vi "创建配方子VI.vi"() -> (3 "配方编号":string)   [LabVIEW 2013]
panel:
  in  "确定":bool
  in  "配方编号":string
  # "请输入配方"
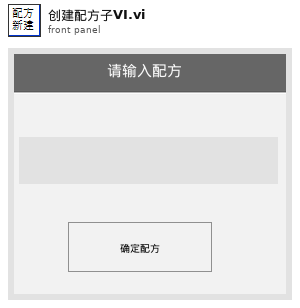
[diagram p1: front panel]
types:
  T1 = enum32{"Invalid", "Standard", "Closed", "Hidden", "Minimized", "Maximized"}
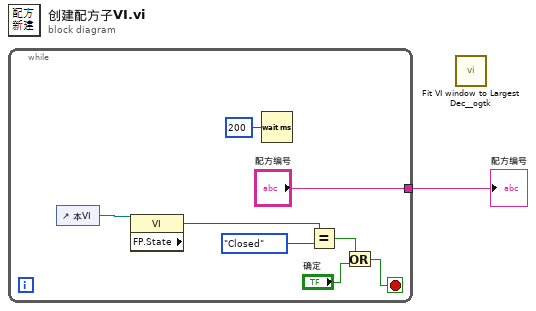
[diagram p0: block diagram]
diagram:
  n1 = while {
    tunnel: ["配方编号"] -> w1
    stop <- w2 stop-if-true
    n2 = control-ref of="本VI"() -> (w4:refnum<vi>)
    n3 = property class="VI"(reference=w4) -> ("FP.State"=w5:T1)  [unwired: 1 in, 2 out]
    n4 = Wait (ms)(milliseconds to wait=u32 200 ("等待时间（毫秒）")) -> ()  [unwired: 1 out]
    n5 = Equal?(x=w5, y=T1."Closed" ("前面板窗口:状态")) -> (x = y?=w7:bool)
    n6 = Or(x=w7, y="确定") -> (x .or. y?=w2:bool)
  }
  "配方编号" <- w1
  n7 = call <userlib>:"Fit VI window to Largest Dec__ogtk.vi"() -> ()  [unwired: 6 in, 2 out]
